vi "Get Setting - Error_Log_Folder.vi"(8 "Error In":errorcluster) -> (0 "Error Out":errorcluster, 3 "Error_Log_Folder":path)   [LabVIEW 2016, in "Error Manager.lvlib" / "Settings.lvclass"]
uses:
  Settings.lvclass
  Settings (class variable).vi
panel:
  # "Input\nInputs to the VI"
  # "Development\nControls or indicators that are useful for development or testing, but which are not outputs of the VI."
  # "Output\nOutputs of the VI"
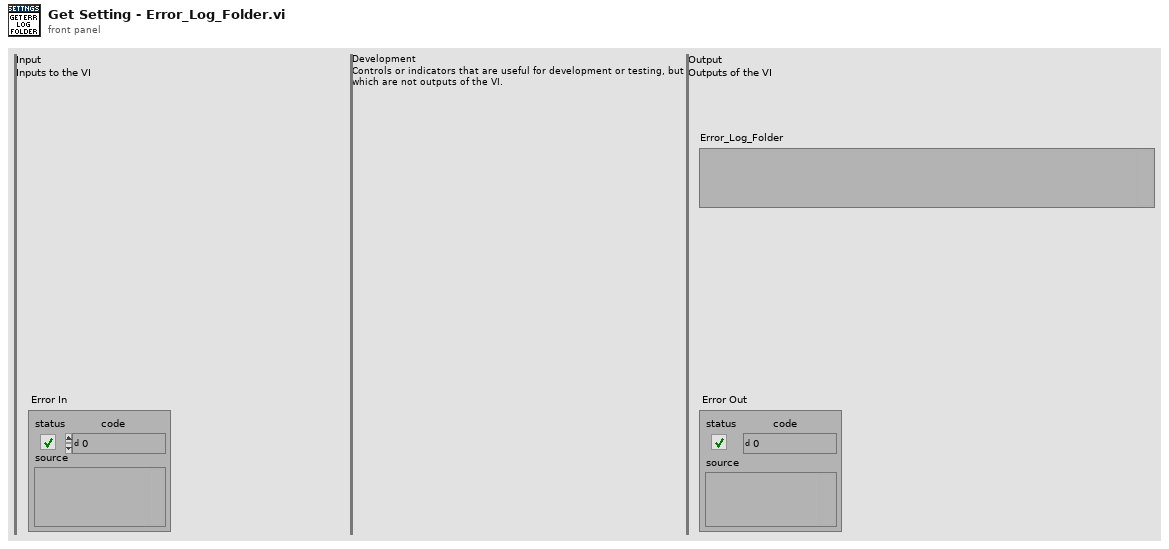
[diagram p1: front panel]
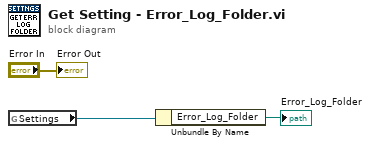
[diagram p0: block diagram]
diagram:
  n1 = global read "Settings (class variable).vi" "Settings"() -> (w1:refnum<class "Settings.lvclass">)
  n2 = Unbundle By Name(w1) -> ("Error_Log_Folder"=→"Error_Log_Folder":path)
  "Error Out" <- "Error In"
